vi "Configure Zone Marker.vi"(0 "VISA resource name":refnum<visa-resource-name>, 1 "Zone Setting (0:Frequency)":i32(ring) items=["Frequency", "Point", "Time", "Relative"], 2 "Marker Type (0:Zoom Marker)":i32(ring) items=["Zone Marker", "Spot Marker"], 3 "Marker (0:Marker 1)":i32(ring) items=["Marker 1", "Marker 2", "Marker 3", "Marker 4", "Marker 5", "Marker 6", "Marker 7", "Marker 8", "Marker 9", "Marker 10"], 5 "Zone Marker Frequency (3000000000Hz)":dbl=3000000000.0 min=-100000000.0 max=43100000000.0, 7 "Point (100)":i32=100 min=0 max=10000, 9 "Zone Marker Time (0.1ms)":dbl=0.1 min=-1000.0 max=1000.0, 11 "error in (no error)":errorcluster, 12 "Zone Width":T1={"Width Frequency (1000000Hz)"=1000000.0, "Width Point (100)"=100, "Width (0:0.5 div)"=0} {"Width (0:0.5 div)" items=["0.5 div", "Spot", "1 div", "2 div", "5 div", "10 div"]; "Width Point (100)" min=1 max=10001}, 13 "Relative Center Frequency (3000000000Hz)":dbl=3000000000.0, 14 "Couple Zone (0:Off)":i32(ring) items=["Off", "On"]) -> (4 "VISA resource name out":refnum<visa-resource-name>, 15 "error out":errorcluster)   [LabVIEW 2023, in "Anritsu Signal Analyzer Series.lvlib"]
doc: "Configures the zone marker settings of the spectrum analyzer."
uses:
  Anritsu Signal Analyzer Series.lvlib
panel:
  # "Hz"
  # "Hz"
  # "ms"
  # "Hz"
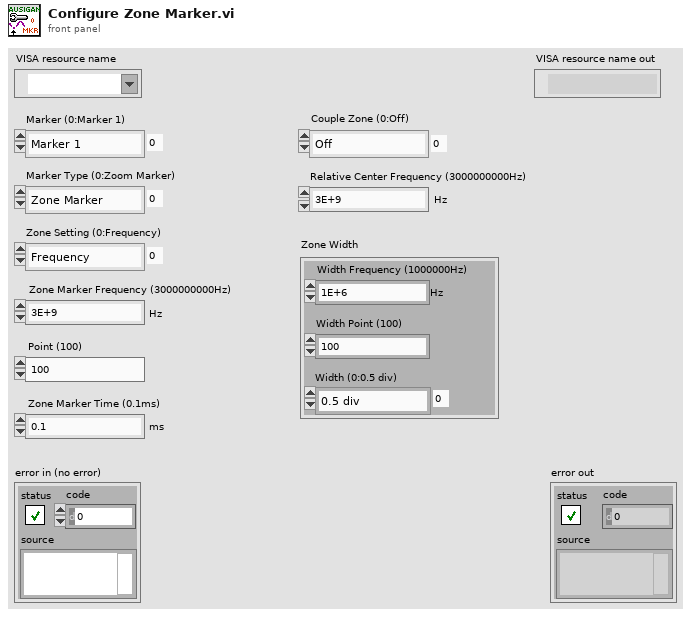
[diagram p1: front panel]
types:
  T1 = cluster{"Width Frequency (1000000Hz)":dbl, "Width Point (100)":i32, "Width (0:0.5 div)":i32}
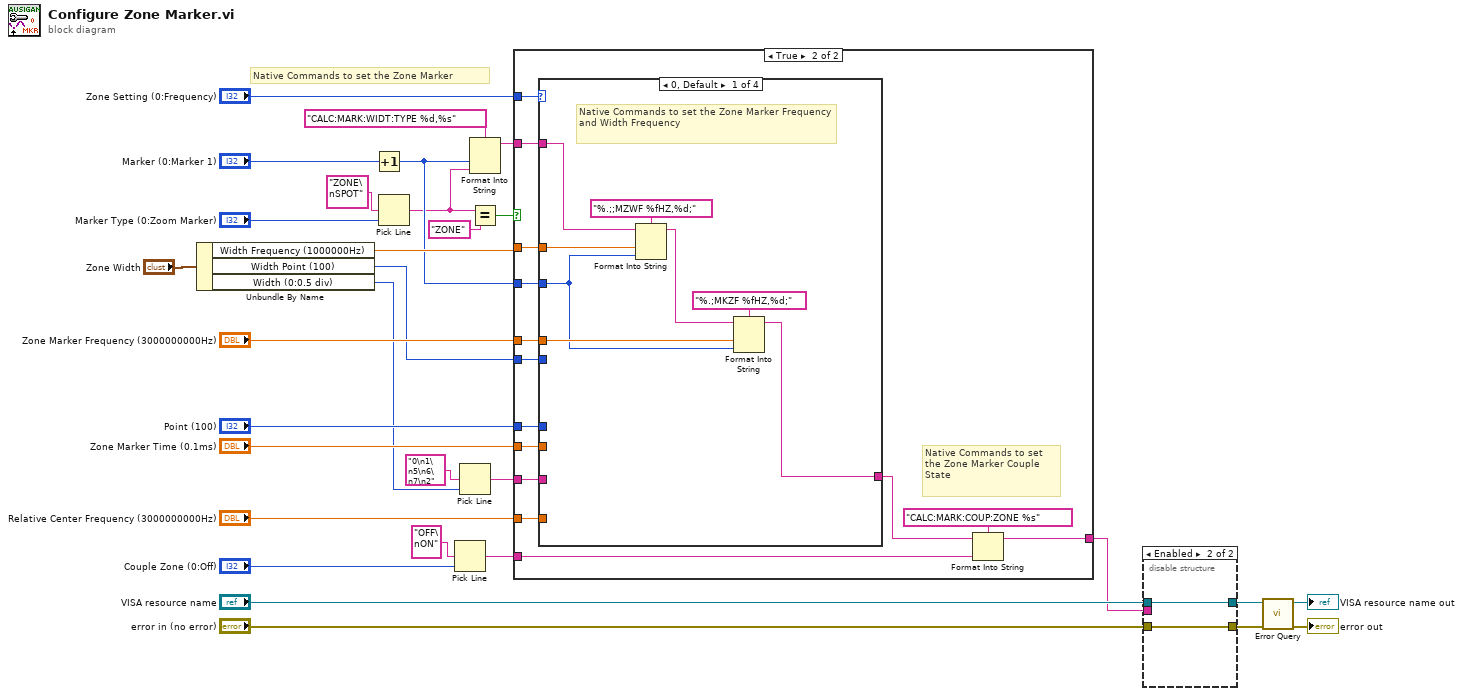
[diagram p0: block diagram]
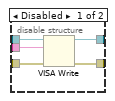
[diagram p2: hidden frame]
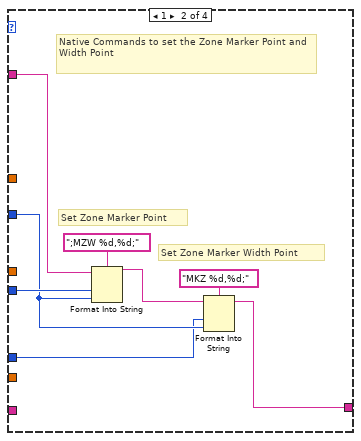
[diagram p4: hidden frame]
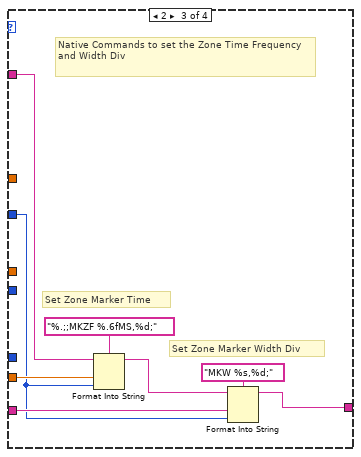
[diagram p5: hidden frame]
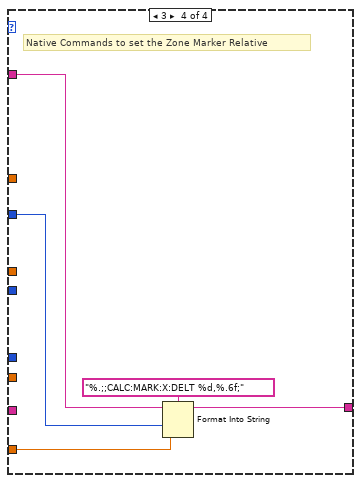
[diagram p6: hidden frame]
diagram:
  # "Native Commands to set the Zone Marker"
  n1 = Unbundle By Name("Zone Width") -> ("Width Frequency (1000000Hz)"=w17:dbl, "Width Point (100)"=w16:i32, "Width (0:0.5 div)"=w15:i32)
  n2 = Increment(x="Marker (0:Marker 1)") -> (x+1=w5:i32)
  n3 = Pick Line(multi-line string="ZONE\nSPOT" ("複数行文字列"), line index="Marker Type (0:Zoom Marker)") -> (output string=w3:string)  [unwired: 1 in]
  n4 = Pick Line(multi-line string="OFF\nON" ("複数行文字列"), line index="Couple Zone (0:Off)") -> (output string=w6:string)  [unwired: 1 in]
  n5 = Pick Line(multi-line string="0\n1\n5\n6\n7\n2" ("複数行文字列"), line index=w15) -> (output string=w1:string)  [unwired: 1 in]
  n6 = Format Into String(format string="CALC:MARK:WIDT:TYPE %d,%s" ("_CommandSet"), w5, w3) -> (resulting string=w11:string)  [unwired: 2 in, 1 out]
  n7 = Equal?(x=w3, y="ZONE" ("_Case0")) -> (x = y?=w12:bool)
  n8 = case shown="True" w12 {
    tunnel: w11 -> [w31 w44]
    tunnel: "Zone Setting (0:Frequency)" -> [_ w45]
    tunnel: w17 -> [_ w43]
    tunnel: w5 -> [_ w42]
    tunnel: "Zone Marker Frequency (3000000000Hz)" -> [_ w41]
    tunnel: w16 -> [_ w40]
    tunnel: "Point (100)" -> [_ w39]
    tunnel: "Zone Marker Time (0.1ms)" -> [_ w38]
    tunnel: w1 -> [_ w37]
    tunnel: "Relative Center Frequency (3000000000Hz)" -> [_ w36]
    tunnel: w6 -> [_ w35]
    tunnel: [w31 w32] -> w8
    frame False {
      # "Native Commands to set the Spot Marker"
    }
    frame True {
      # "Native Commands to set the Zone Marker Couple State"
      n9 = case shown="0, Default" w45 {
        tunnel: w44 -> [w51 w59 w63 w72]
        tunnel: w43 -> [w53 _ _ _]
        tunnel: w42 -> [w47 w56 w65 w70]
        tunnel: w41 -> [w50 _ _ _]
        tunnel: w40 -> [_ w61 _ _]
        tunnel: w39 -> [_ w54 _ _]
        tunnel: w38 -> [_ _ w69 _]
        tunnel: w37 -> [_ _ w67 _]
        tunnel: w36 -> [_ _ _ w73]
        tunnel: [w46 w55 w62 w71] -> w33
        frame 0, Default {
          # "Native Commands to set the Zone Marker Frequency and Width Frequency"
          n10 = Format Into String(format string="%.;;MZWF %fHZ,%d;" ("Format String"), initial string=w51, w53, w47) -> (resulting string=w49:string)  [unwired: 1 in, 1 out]
          n11 = Format Into String(format string="%.;MKZF %fHZ,%d;" ("Format String"), initial string=w49, w50, w47) -> (resulting string=w46:string)  [unwired: 1 in, 1 out]
        }
        frame 1 {
          # "Native Commands to set the Zone Marker Point and Width Point"
          # "Set Zone Marker Width Point"
          # "Set Zone Marker Point"
          n12 = Format Into String(format string=";MZW %d,%d;" ("Format String"), initial string=w59, w61, w56) -> (resulting string=w57:string)  [unwired: 1 in, 1 out]
          n13 = Format Into String(format string="MKZ %d,%d;" ("Format String"), initial string=w57, w54, w56) -> (resulting string=w55:string)  [unwired: 1 in, 1 out]
        }
        frame 2 {
          # "Native Commands to set the Zone Time Frequency and Width Div"
          # "Set Zone Marker Time"
          # "Set Zone Marker Width Div"
          n14 = Format Into String(format string="%.;;MKZF %.6fMS,%d;" ("Format String"), initial string=w63, w69, w65) -> (resulting string=w66:string)  [unwired: 1 in, 1 out]
          n15 = Format Into String(format string="MKW %s,%d;" ("_CommandSet"), initial string=w66, w67, w65) -> (resulting string=w62:string)  [unwired: 1 in, 1 out]
        }
        frame 3 {
          # "Native Commands to set the Zone Marker Relative"
          n16 = Format Into String(format string="%.;;CALC:MARK:X:DELT %d,%.6f;" ("_CommandSet"), initial string=w72, w70, w73) -> (resulting string=w71:string)  [unwired: 1 in, 1 out]
        }
      }
      n17 = Format Into String(format string="CALC:MARK:COUP:ZONE %s" ("_CommandSet"), initial string=w33, w35) -> (resulting string=w32:string)  [unwired: 1 in, 1 out]
    }
  }
  n18 = disable-structure shown="Enabled" {
    disable-tunnel: "VISA resource name" -> [w79 w81]
    disable-tunnel: "error in (no error)" -> [w78 w80]
    disable-tunnel: [w77 w81] -> w10
    disable-tunnel: [w76 w80] -> w9
    disable-tunnel: w8 -> [w75 _]
    frame Disabled {
      n19 = VISA Write(VISA resource name=w79, write buffer=w75, error in (no error)=w78) -> (VISA resource name out=w77:refnum<visa-resource-name>, error out=w76:errorcluster)  [unwired: 1 out]
    }
    frame Enabled {
    }
  }
  n20 = call "Error Query.vi"("error in (no error)"=w9, "VISA resource name"=w10) -> ("error out"=→"error out":errorcluster, "VISA resource name out"=→"VISA resource name out":refnum<visa-resource-name>)  [unwired: 6 in, 2 out]
